vi "ICRA2024测试椭圆分裂 - 副本.vi"() -> ()   [LabVIEW 2018]
doc: "Demonstrates the use of the Network Streams functions to send LED status to the myRIO target."
uses:
  <vilib>/vision/Contour.llb/IMAQ Contour Curve Extraction.ctl
  <vilib>/ErrorRing/Error Ring.xnode
  <vilib>/vision/NI_Vision_Development_Module.lvlib
panel:
  out "len3":dbl
  out "len2":dbl
  out "len1":dbl
  out "len0":dbl
  out "Y4":sgl
  out "Y3":sgl
  out "Y2":sgl
  out "Y1":sgl
  out "Y0":sgl
  in  "Search Rect (entire image)":T1={"Left"=200, "Top"=120, "Right"=2000, "Bottom"=1920, "Rotation"=0.0} {"Rotation" format="%.2f"; "Left" scale=0.0..1024.0; "Right" scale=0.0..1024.0}
  out "长度":dbl
  out "备用的椭圆角度":sgl
  in  "打开轨迹":bool
  out "Image 9":T2(plugin-control)
  in  "Search Direction":T3(ring)
  in  "Contour Selection":T4(ring)
  in  "Number of Erosion":i32=10
  in  "椭圆磁场开关":bool=TRUE
  out "Image 7":T2(plugin-control)
  out "Ellipse":T5 {"Center"."Y" format="%.2f"; "Center"."X" format="%.2f"}
  out "Image 5":T2(plugin-control)
  in  "Contour Points Settings":T6={"Overlay?"=FALSE, "Color"=16711680, "Width"=1, "Maintain Width?"=TRUE}
  in  "Contour Equation Settings":T6={"Overlay?"=TRUE, "Color"=3381759, "Width"=1, "Maintain Width?"=TRUE}
  out "ROI Descriptor Out":T7 {"Contours"."Type" items=["No Selection", "Point", "Line", "Rectangle", "Oval", "Polygon", "Freehand Region", "Annulus", "Unused2", "Unused3", "Broken Line", "Freehand Line", "Rotated Rectangle"]}
  in  "Curve Extraction":T8={"Extraction Mode"=0, "Edge Threshold"=75, "Edge Filter Size"=1, "Min Length"=25, "Search Step Size"=15, "Max Endpoint Gap"=10, "Subpixel"=TRUE} {"Extraction Mode" items=["Normal", "Uniform Regions"]; "Edge Filter Size" items=["Fine", "Normal", "Contour Tracing"]; "Max Endpoint Gap" min=0; "Search Step Size" min=1 max=255 step=1; "Min Length" min=0; "Edge Threshold" min=1 max=350 step=1}
  out "Image 4":T2(plugin-control)
  out "Image":T2(plugin-control)
  in  "Acquisition Control::Acquisition Frame Rate":dbl=19.50304412841797 min=1.4211589097976685 max=44.94382095336914
  out "Stopped":bool
  in  "Stop (F) 2":bool caption="Stop (F)"
  out "Objects 2":T9(array[cluster]) {"Aspect Ratio" format="%.2f"; "Orientation" format="%.2f"; "Area" format="%.2f"; "Object Center"."Y" format="%.2f"; "Object Center"."X" format="%.2f"}
  in  "Settings 2":T10={"Objects"=0, "Threshold"=128, "Reject Border"=FALSE, "Fill Holes"=FALSE, "Min Object Size"=TRUE, "Min Size"=20000, "Max Object Size"=FALSE, "Max Size"=100, "Show Search Area"=FALSE, "Show Center"=TRUE, "Show Bounding Box"=TRUE} {"Objects" items=["Bright Objects", "Dark Objects"]; "Threshold" min=1 max=999999999 step=1; "Max Size" min=1 max=999999999 step=1; "Min Size" min=1 max=999999999 step=1}
  in  "Range 2":cluster{"Lower value":sgl, "Upper value":sgl}={"Lower value"=0.0, "Upper value"=230.0} {"Upper value" format="%.2f"; "Lower value" format="%.2f"}
  in  "Pause":bool
  out "Array":dbl[](array[numeric])
  in  "Parameter Settings":T11(tab)=enum."Ribbon Oscillating Field" caption="Field Types"
  in  "fg":dbl
  in  "pg":dbl
  in  "dg":dbl
  in  "Ag":dbl
  in  "AoOF":dbl
  in  "fo":sgl
  in  "do":sgl
  in  "oo":sgl
  in  "po":sgl
  in  "cc":sgl
  in  "pc":sgl
  in  "wc":sgl
  in  "dc":sgl
  in  "Ac":dbl
  in  "pr":sgl
  in  "Ar":dbl=8.0
  in  "wr":sgl=18.0
  in  "dr":sgl
  in  "Dis phase step":dbl
  in  "Dis phase frequency (Hz)":dbl
  in  "Dis tumbling frequency (Hz)":dbl
  in  "Dis strength(mT)":dbl
  in  "Swa strength (mT)":dbl
  in  "Swa frequency (Hz)":dbl
  in  "Swa pitch angle (deg)":dbl
  in  "Swa direction angle (deg)":dbl
  in  "Swa ratio":dbl=1.0
  in  "Pitch Angle (rotating around Constant, deg)":dbl
  in  "Ratio (A/C)":sgl=3.0
  in  "Direction Angle (deg)":sgl=90.0
  in  "Pitch Angle (rotating around Origin, deg)":sgl
  in  "Frequency (Hz)":sgl=6.0
  in  "Strength (mT)":dbl=3.0
  in  "Ar 2":dbl=5.0 caption="Ar"
  in  "ratio":sgl=1.0
  in  "运动方向":sgl
  in  "长轴方向":sgl
  in  "wr  2":sgl=8.0
  in  "速度大小":sgl
  out "Angle":dbl
  out "aspect ratio":dbl
  out "时间":i32
  out "Numeric 5":i32
  in  "Stop":bool
  out "error out":errorcluster
  in  "Target IP Address":string="172.22.11.2"
  # "Overview: Magnetic field calculation, and send parameters to myRIO\nInstructions:\n1. Verify the value of Target IP Address. Set Visa resource name.\n2. Ensure RT Main.vi is already running. \n3. Run this VI. Set parameters of magnetic field."
  # "Strength (mT)"
  # "Pitch Angle (deg)"
  # "Direction Angle (deg)"
  # "Frequency (Hz)"
  # "Strength (mT)"
  # "Oscilation Frequency (Hz)"
  # "Oscilation Angle (deg)"
  # "Pitch Angle (deg)"
  # "Direction Angle (deg)"
  # "Strength (mT)"
  # "Frequency (Hz)"
  # "Pitch Angle (deg)"
  # "Direction Angle (deg)"
  # "Conical Angle (deg)"
  # "Strength (mT)"
  # "Frequency (Hz)"
  # "Pitch Angle (deg)"
  # "Direction Angle (deg)"
  # "Strength (mT)"
  # "Tumbling Frequency (Hz)"
  # "Phase Frequency (Hz)"
  # "Phase Step"
  # "Strength (mT)"
  # "Frequency (Hz)"
  # "Pitch Angle (deg)"
  # "Direction Angle (deg)"
  # "Ratio"
  # "Strength (mT)"
  # "Frequency (Hz)"
  # "Ratio (A/C)"
  # "Direction Angle (deg)"
  # "Pitch Angle (rotating around Origin, deg)"
  # "Pitch Angle (rotating around Constant, deg)"
  # "Strength (mT)"
  # "Frequency (Hz)"
  # "Pitch Angle  (deg)"
  # "longaxis"
  # "Direction Angle (deg)"
  # "ratio (l/s)"
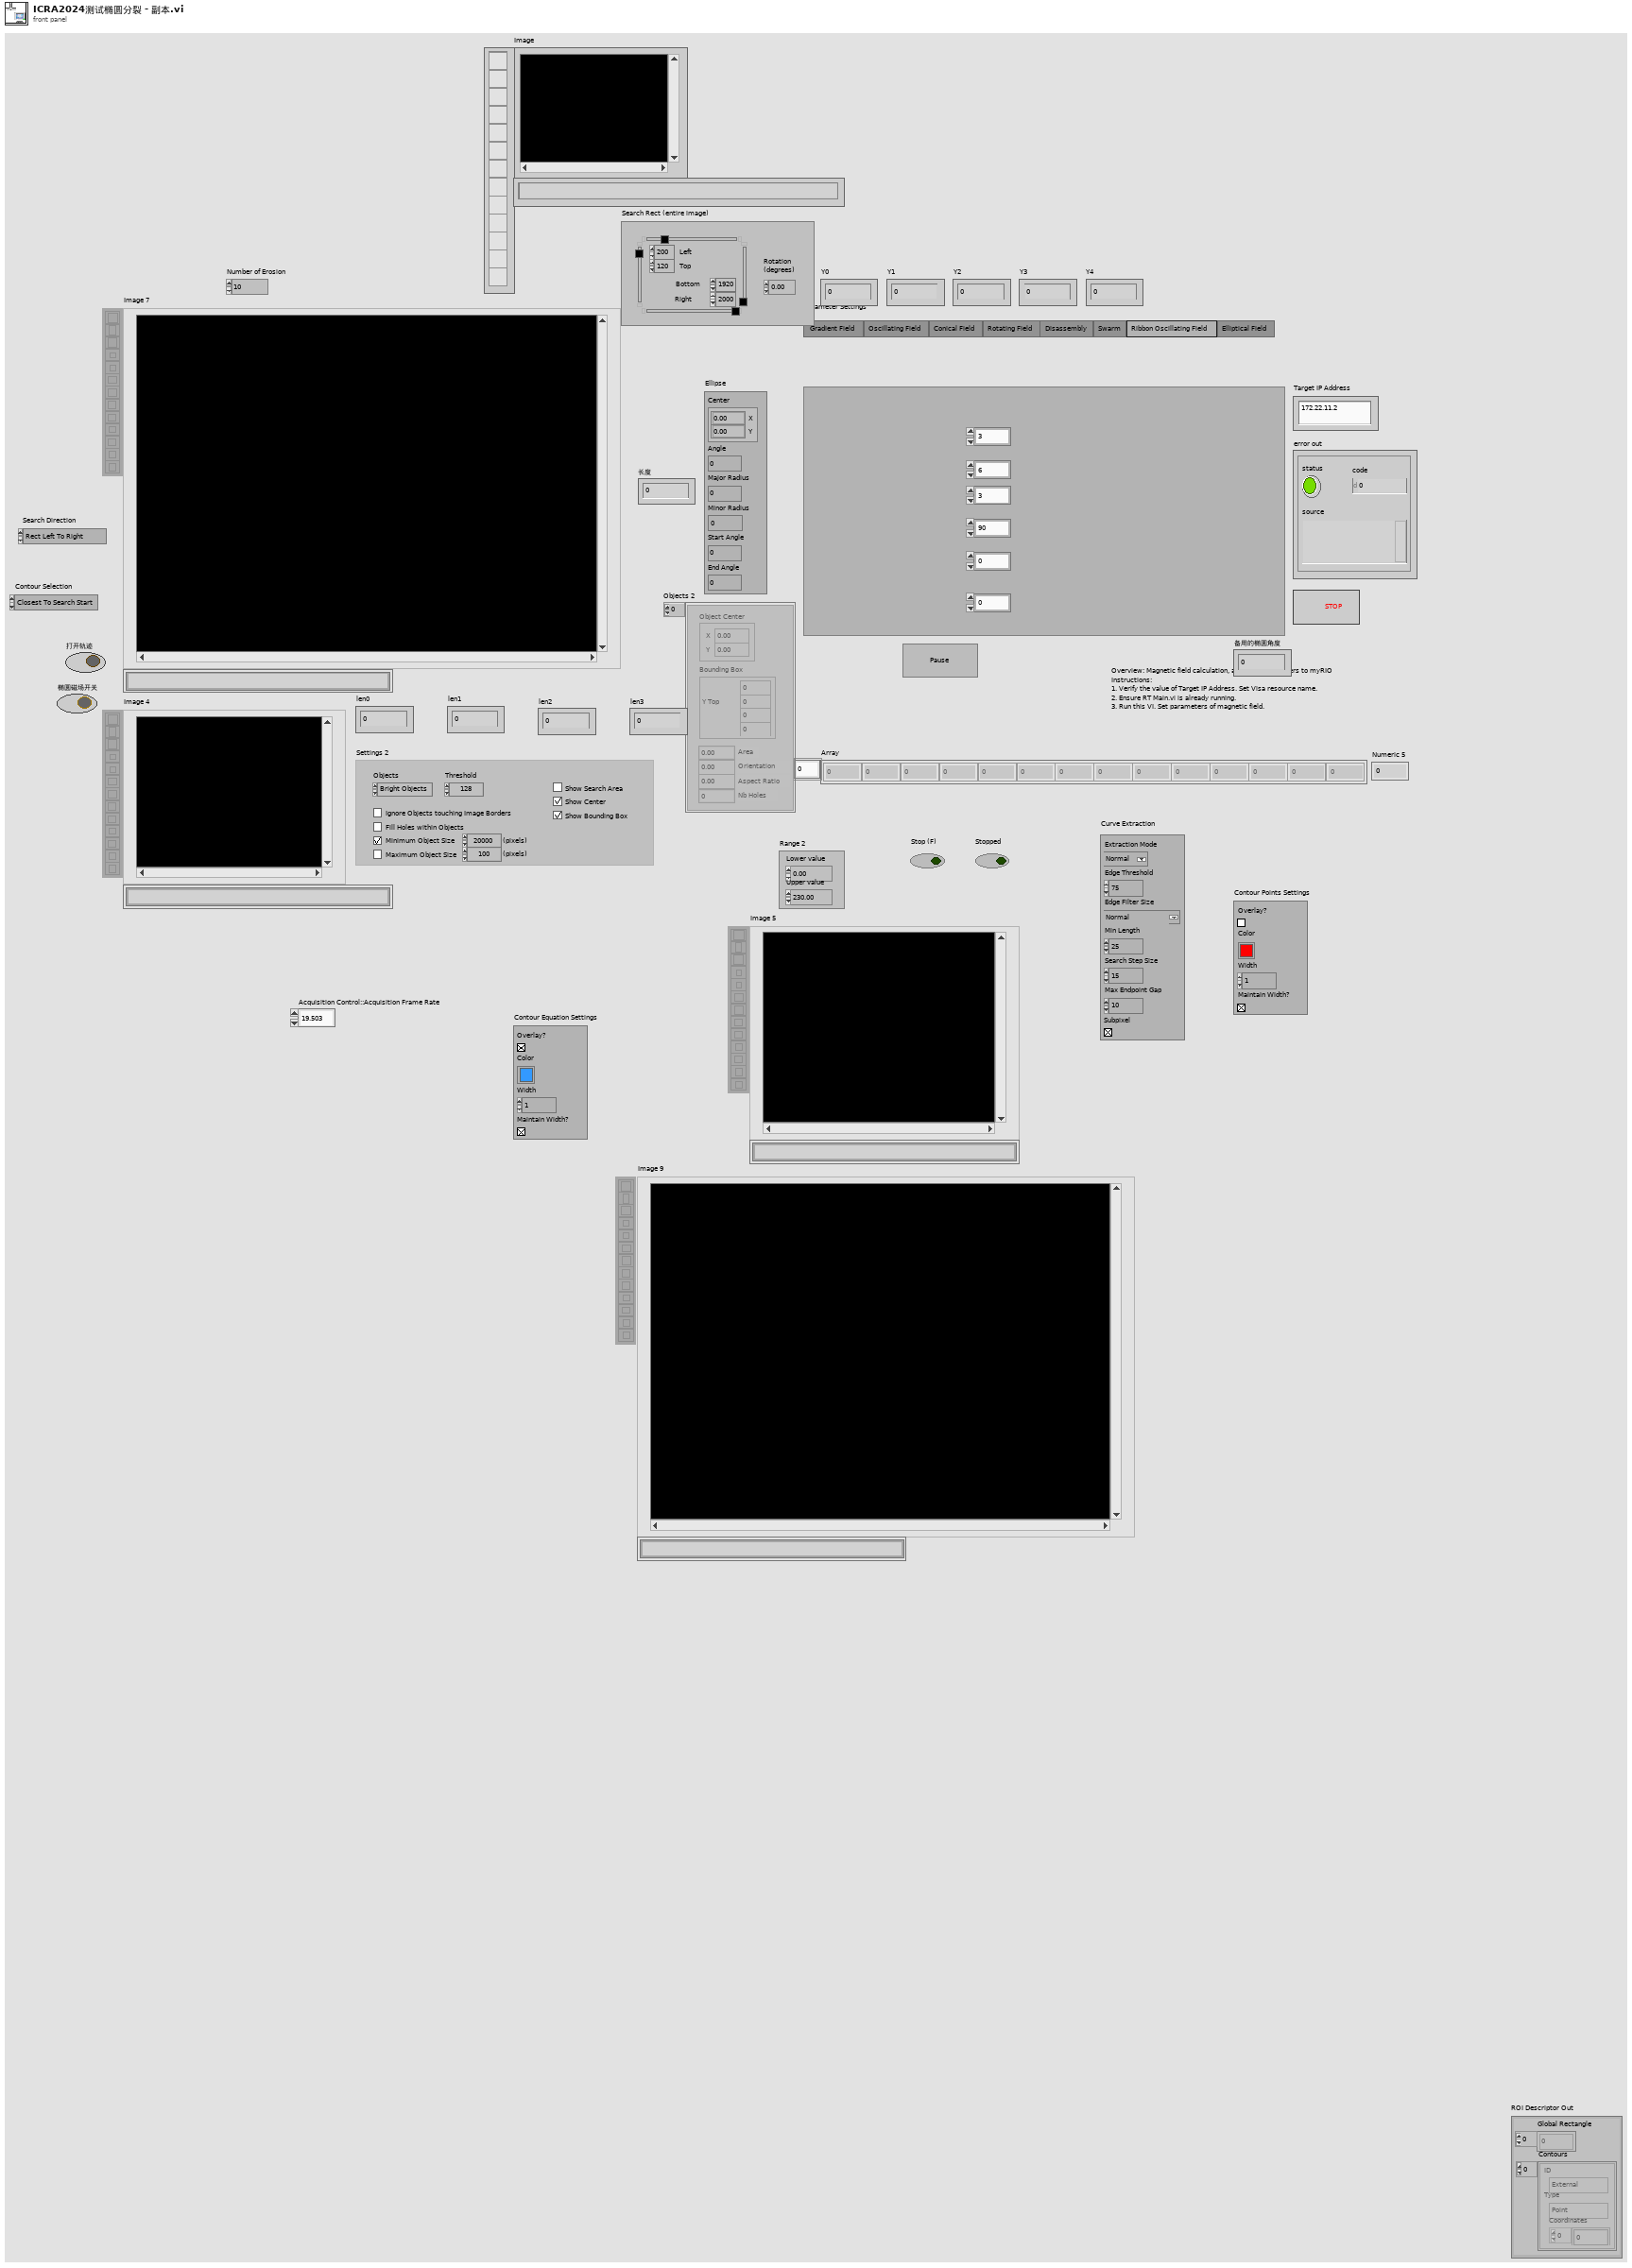
[diagram p1: front panel]
types:
  T1 = typedef "IMAQ Rectangle" = cluster{"Left":i32, "Top":i32, "Right":i32, "Bottom":i32, "Rotation":dbl}
  T2 = typedef "IMAQ Image.ctl" = refnum<image>
  T3 = enum16{"Rect Left To Right", "Rect Right To Left", "Rect Top To Bottom", "Rect Bottom To Top", "Annulus Inner To Outer", "Annulus Outer To Inner", "Annulus Start Angle To End Angle", "Annulus End Angle To Start Angle"}
  T4 = enum16{"Closest To Search Start", "Maximum Length", "Strongest Mean Gradient Change"}
  T5 = cluster{"Center":cluster{"X":sgl, "Y":sgl}, "Angle":dbl, "Major Radius":dbl, "Minor Radius":dbl, "Start Angle":dbl, "End Angle":dbl}
  T6 = cluster{"Overlay?":bool, "Color":u32, "Width":u32, "Maintain Width?":bool}
  T7 = typedef "ROI Descriptor" = cluster{"Global Rectangle":i32[], "Contours":cluster{"ID":enum32{"External", "Internal"}, "Type":u32, "Coordinates":i32[]}[]}
  T8 = typedef "IMAQ Contour Curve Extraction.ctl" = cluster{"Extraction Mode":u32, "Edge Threshold":i32, "Edge Filter Size":u32, "Min Length":i32, "Search Step Size":i32, "Max Endpoint Gap":i32, "Subpixel":bool}
  T9 = cluster{"Object Center":cluster{"X":sgl, "Y":sgl}, "Bounding Box":cluster{"X Left":i32, "Y Top":i32, "X Right":i32, "Y Bottom":i32}, "Area":sgl, "Orientation":sgl, "Aspect Ratio":sgl, "Nb Holes":i32}[]
  T10 = cluster{"Objects":u16, "Threshold":i32, "Reject Border":bool, "Fill Holes":bool, "Min Object Size":bool, "Min Size":i32, "Max Object Size":bool, "Max Size":i32, "Show Search Area":bool, "Show Center":bool, "Show Bounding Box":bool}
  T11 = enum32{"Gradient Field ", "Oscillating Field", "Conical Field", "Rotating Field", "Disassembly", "Swarm", "Ribbon Oscillating Field", "Elliptical Field"}
  T12 = enum32{"AutoM", "Close", "Dilate", "Erode", "Gradient", "Gradient in", "Gradient out", "HitMiss", "Open", "PClose", "POpen", "Thick", "Thin"}
  T13 = typedef "Image Type" = u32
  T14 = cluster{"Objects[0]":cluster{"Object Center":cluster{"X":sgl, "Y":sgl}, "Bounding Box":cluster{"X Left":i32, "Y Top":i32, "X Right":i32, "Y Bottom":i32}, "Area":sgl, "Orientation":sgl, "Aspect Ratio":sgl, "Nb Holes":i32}, "Objects[1]":cluster{"Object Center":cluster{"X":sgl, "Y":sgl}, "Bounding Box":cluster{"X Left":i32, "Y Top":i32, "X Right":i32, "Y Bottom":i32}, "Area":sgl, "Orientation":sgl, "Aspect Ratio":sgl, "Nb Holes":i32}, "Objects[2]":cluster{"Object Center":cluster{"X":sgl, "Y":sgl}, "Bounding Box":cluster{"X Left":i32, "Y Top":i32, "X Right":i32, "Y Bottom":i32}, "Area":sgl, "Orientation":sgl, "Aspect Ratio":sgl, "Nb Holes":i32}, "Objects[3]":cluster{"Object Center":cluster{"X":sgl, "Y":sgl}, "Bounding Box":cluster{"X Left":i32, "Y Top":i32, "X Right":i32, "Y Bottom":i32}, "Area":sgl, "Orientation":sgl, "Aspect Ratio":sgl, "Nb Holes":i32}, "Objects[4]":cluster{"Object Center":cluster{"X":sgl, "Y":sgl}, "Bounding Box":cluster{"X Left":i32, "Y Top":i32, "X Right":i32, "Y Bottom":i32}, "Area":sgl, "Orientation":sgl, "Aspect Ratio":sgl, "Nb Holes":i32}, "Objects[5]":cluster{"Object Center":cluster{"X":sgl, "Y":sgl}, "Bounding Box":cluster{"X Left":i32, "Y Top":i32, "X Right":i32, "Y Bottom":i32}, "Area":sgl, "Orientation":sgl, "Aspect Ratio":sgl, "Nb Holes":i32}, "Objects[6]":cluster{"Object Center":cluster{"X":sgl, "Y":sgl}, "Bounding Box":cluster{"X Left":i32, "Y Top":i32, "X Right":i32, "Y Bottom":i32}, "Area":sgl, "Orientation":sgl, "Aspect Ratio":sgl, "Nb Holes":i32}, "Objects[7]":cluster{"Object Center":cluster{"X":sgl, "Y":sgl}, "Bounding Box":cluster{"X Left":i32, "Y Top":i32, "X Right":i32, "Y Bottom":i32}, "Area":sgl, "Orientation":sgl, "Aspect Ratio":sgl, "Nb Holes":i32}, "Objects[8]":cluster{"Object Center":cluster{"X":sgl, "Y":sgl}, "Bounding Box":cluster{"X Left":i32, "Y Top":i32, "X Right":i32, "Y Bottom":i32}, "Area":sgl, "Orientation":sgl, "Aspect Ratio":sgl, "Nb Holes":i32}}
  T15 = cluster{"Object Center":cluster{"X":sgl, "Y":sgl}, "Bounding Box":cluster{"X Left":i32, "Y Top":i32, "X Right":i32, "Y Bottom":i32}, "Area":sgl, "Orientation":sgl, "Aspect Ratio":sgl, "Nb Holes":i32}
  T16 = cluster{"X Left":i32, "Y Top":i32, "X Right":i32, "Y Bottom":i32}
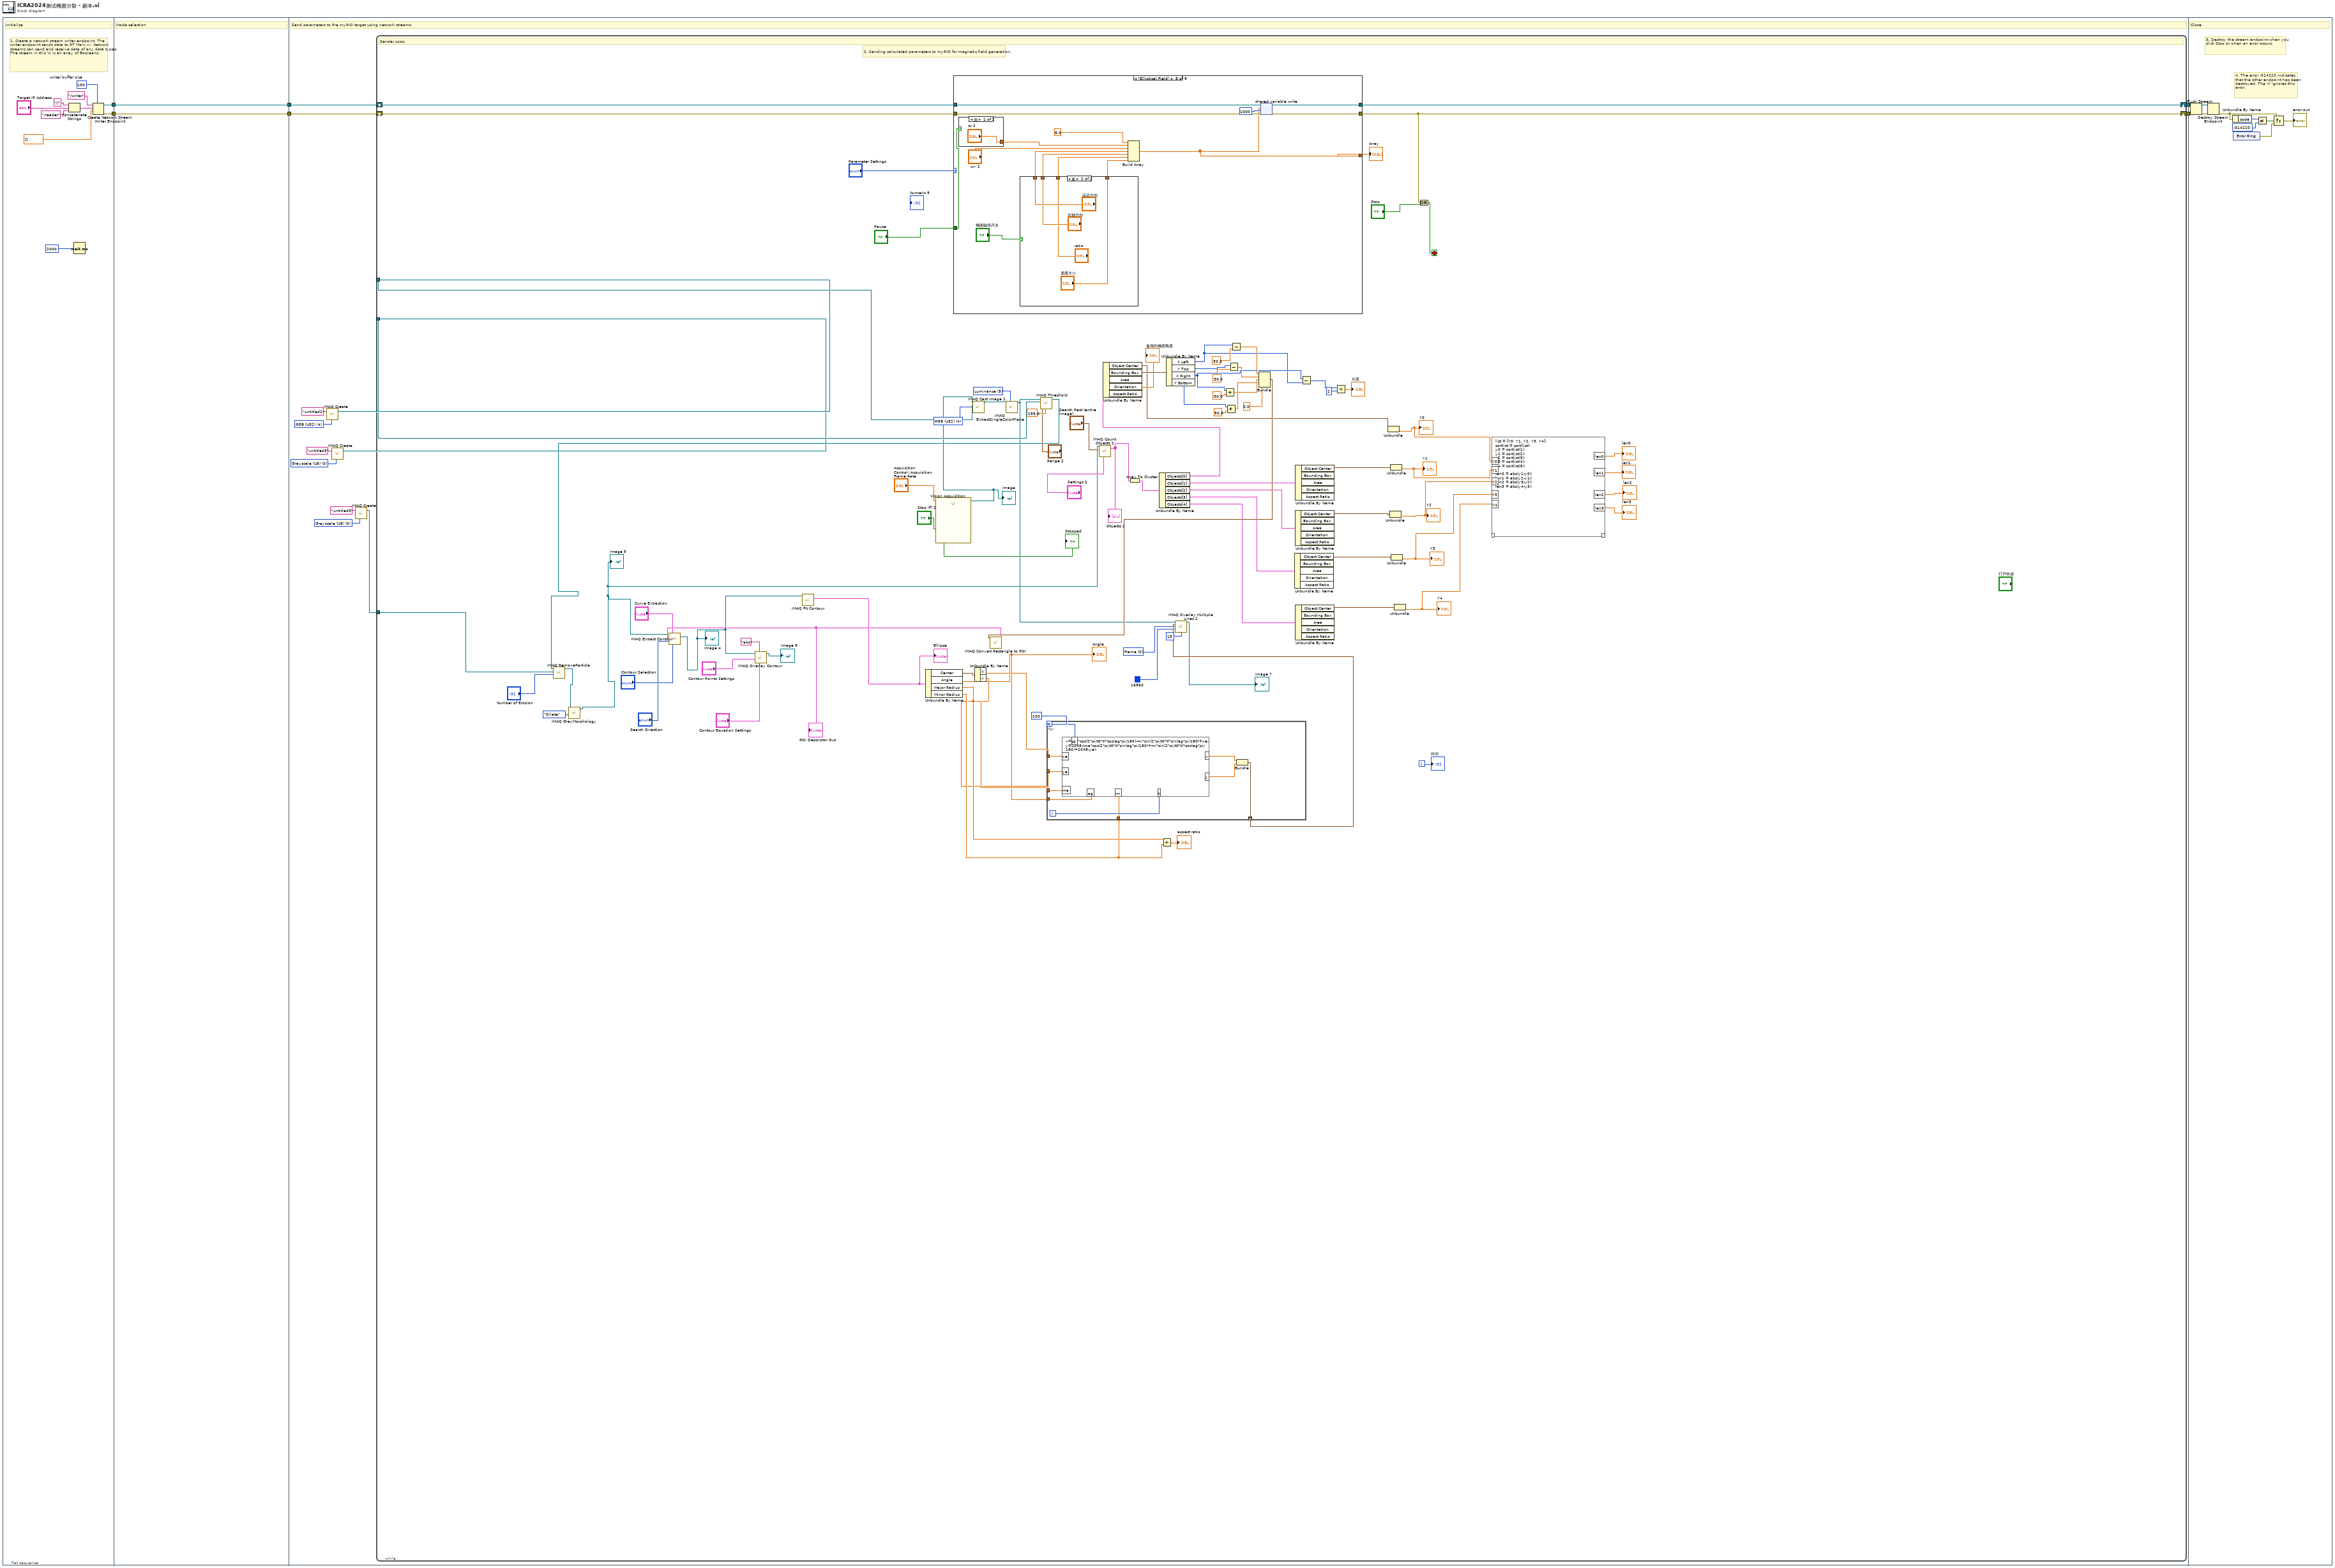
[diagram p0: block diagram]
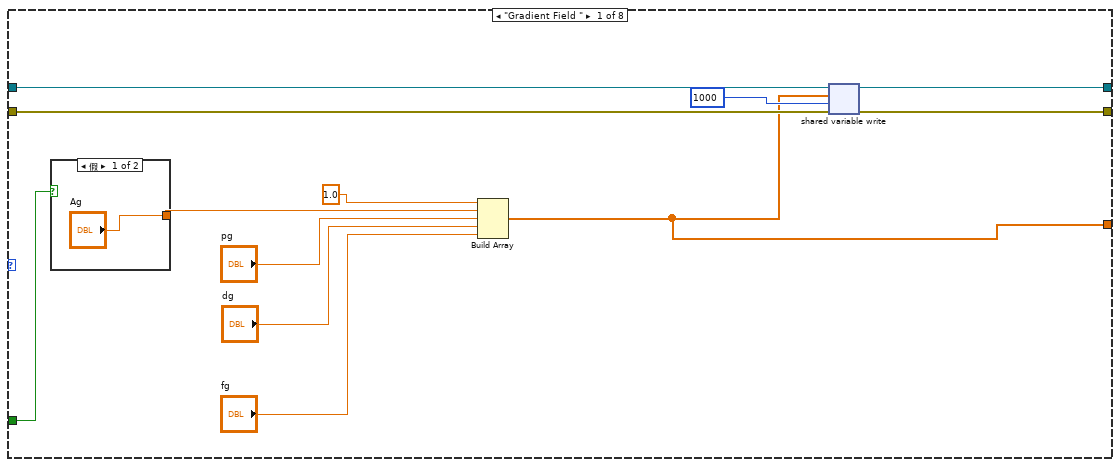
[diagram p2: hidden frame]
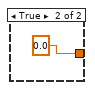
[diagram p3: hidden frame]
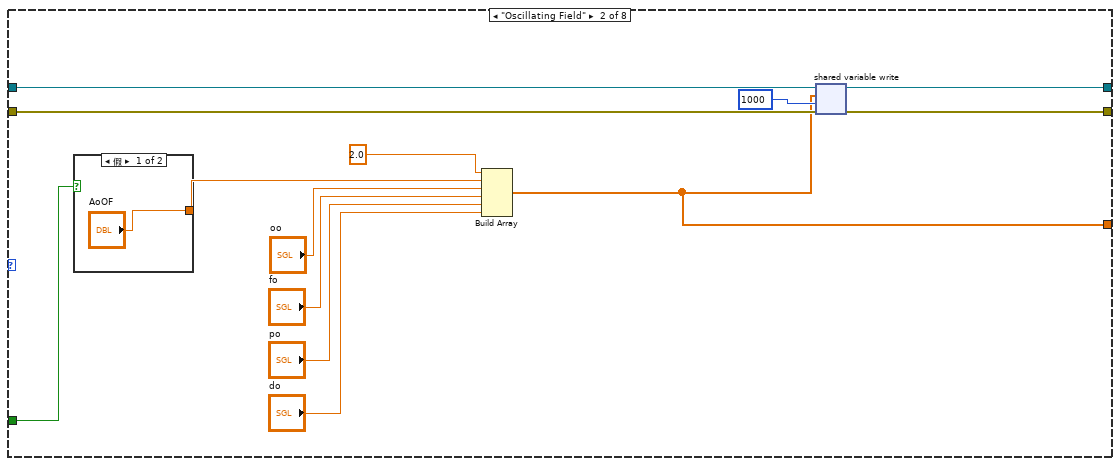
[diagram p4: hidden frame]
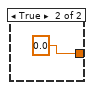
[diagram p5: hidden frame]
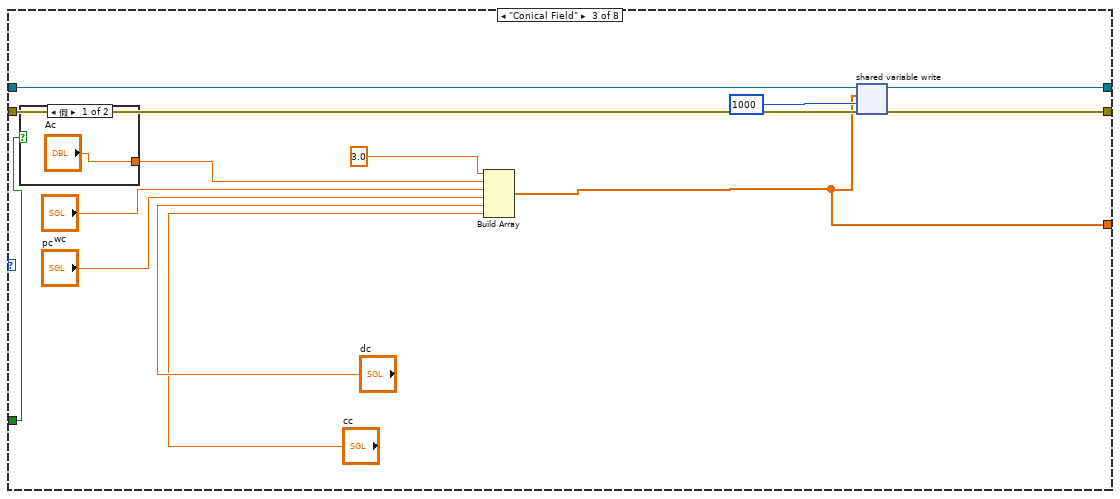
[diagram p6: hidden frame]
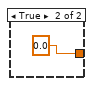
[diagram p7: hidden frame]
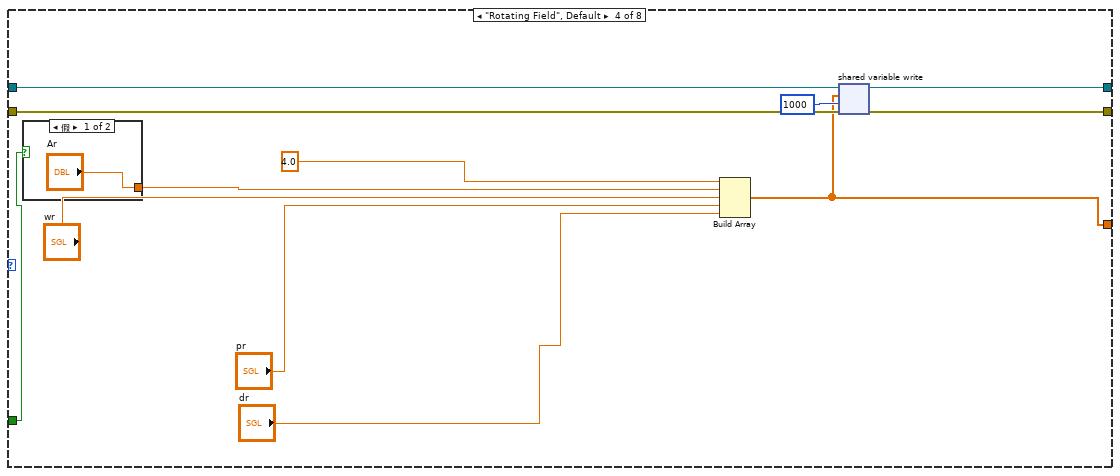
[diagram p8: hidden frame]
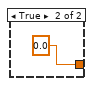
[diagram p9: hidden frame]
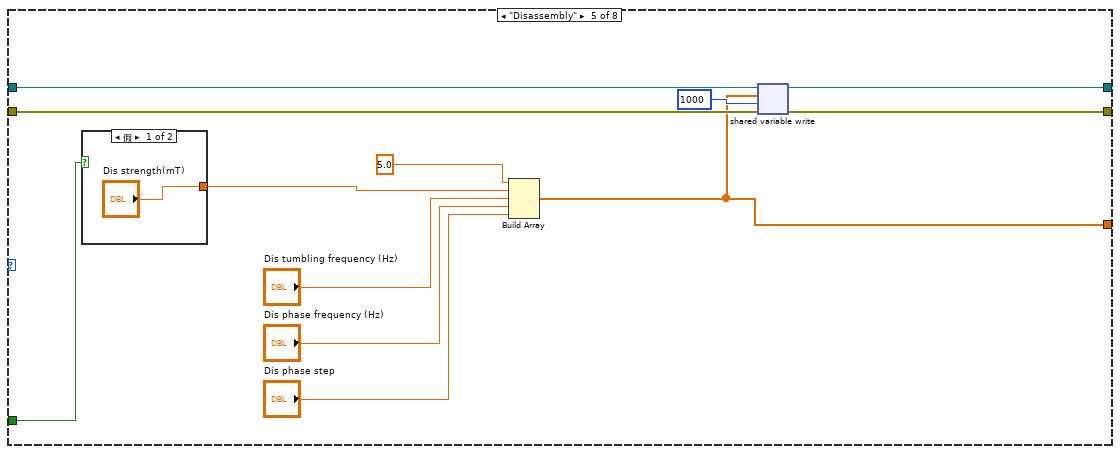
[diagram p10: hidden frame]
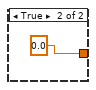
[diagram p11: hidden frame]
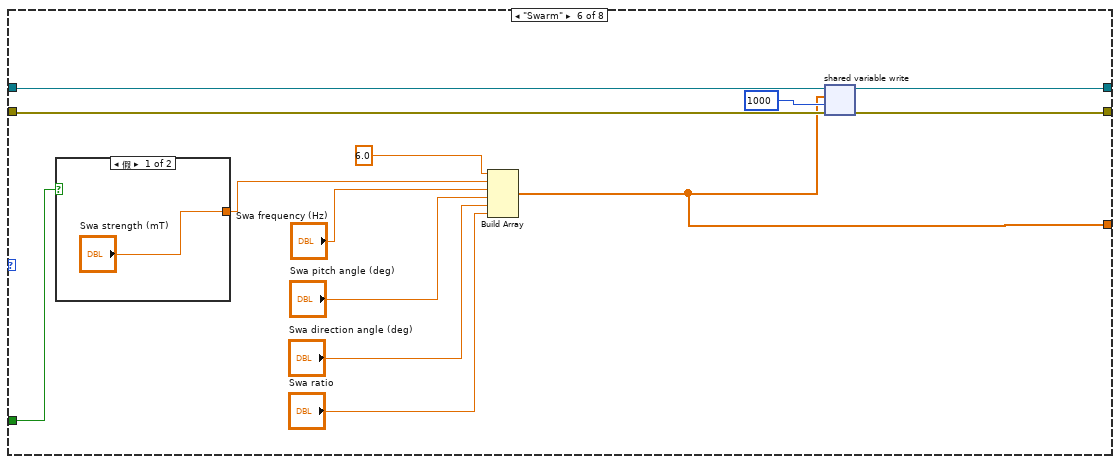
[diagram p12: hidden frame]
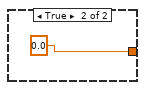
[diagram p13: hidden frame]
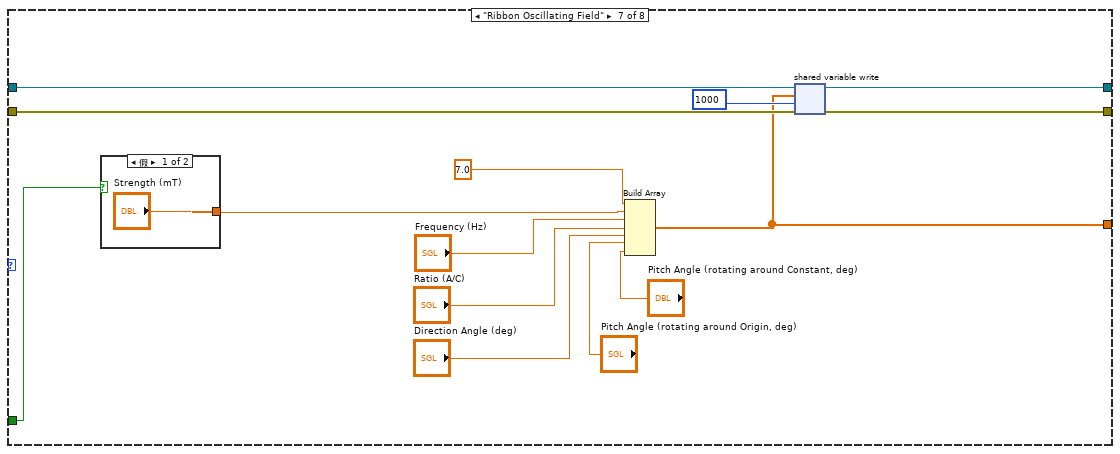
[diagram p14: hidden frame]
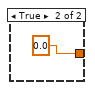
[diagram p15: hidden frame]
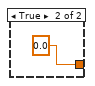
[diagram p17: hidden frame]
diagram:
  n1 = flat-sequence {
    tunnel: [w11] -> w2
    tunnel: [w10] -> w1
    tunnel: [w18] -> w4
    tunnel: [w17] -> w3
    tunnel: w1 -> [w17]
    tunnel: w2 -> [w18]
    tunnel: [w29] -> w6
    tunnel: w4 -> [w31]
    tunnel: [w28] -> w5
    tunnel: w3 -> [w30]
    tunnel: w6 -> [w268]
    tunnel: w5 -> [w265]
    frame #0 {
      w9 = 100  # writer buffer size
      # "1. Create a network stream writer endpoint. The writer endpoint sends data to RT Main.vi. Network streams can send and receive data of any data types. The stream in this VI is an array of Booleans."
      # "Initialize"
      n2 = Concatenate Strings("//", "Target IP Address", "/reader") -> (w16:string)
      n3 = Wait (ms)(milliseconds to wait=2000) -> ()  [unwired: 1 out]
      n4 = Create Network Stream Writer Endpoint(7:w9, 9:dbl[] [], 10:w16, 11:"/writer" ("reader name")) -> (0:w10:errorcluster, 3:w11:refnum<k21>)  [unwired: 3 in]
    }
    frame #1 {
      # "Mode selection"
    }
    frame #2 {
      w20 = T13 0 items=["Grayscale (U8)", "Grayscale (I16)", "Grayscale (SGL)", "Complex (CSG)", "RGB (U32)", "HSL (U32)", "RGB (U64)", "Grayscale (U16)"] ("Image Type")
      w24 = T13 0 items=["Grayscale (U8)", "Grayscale (I16)", "Grayscale (SGL)", "Complex (CSG)", "RGB (U32)", "HSL (U32)", "RGB (U64)", "Grayscale (U16)"] ("Image Type")
      w26 = T13 4 items=["Grayscale (U8)", "Grayscale (I16)", "Grayscale (SGL)", "Complex (CSG)", "RGB (U32)", "HSL (U32)", "RGB (U64)", "Grayscale (U16)"] ("Image Type")
      # "Send parameters to the myRIO target using network streams"
      n5 = call "IMAQ Create"("Image Name"="untitled2", "Image Type"=w26) -> ("New Image"=w23:T2)  [unwired: 3 in, 1 out]
      n6 = call "IMAQ Create"("Image Name"="untitled3", "Image Type"=w24) -> ("New Image"=w22:T2)  [unwired: 3 in, 1 out]
      n7 = call "IMAQ Create"("Image Name"="untitled3", "Image Type"=w20) -> ("New Image"=w19:T2)  [unwired: 3 in, 1 out]
      n8 = while {
        shift-right: [w120] -> w28
        shift-left: w30 -> [w122]
        shift-right: [w121] -> w29
        shift-left: w31 -> [w123]
        tunnel: w22 -> [w111]
        tunnel: w23 -> [w106]
        tunnel: w19 -> [w74]
        i -> [w57]
        stop <- w110 stop-if-true
        w93 = u32 0 items=["Frame", "Fill"] ("Drawing Mode (Frame)")
        w105 = T13 4 items=["Grayscale (U8)", "Grayscale (I16)", "Grayscale (SGL)", "Complex (CSG)", "RGB (U32)", "HSL (U32)", "RGB (U64)", "Grayscale (U16)"] ("Image Type")
        w116 = 5 items=["Red", "Green", "Blue", "Hue", "Saturation", "Luminance", "Value", "Intensity"] ("Color Plane")
        # "2. Sending calculated parameters to myRIO for magnetic field generation."
        # "Sender Loop"
        n9 = call "Vision Acquisition"("Acquisition Control::Acquisition Frame Rate"="Acquisition Control::Acquisition Frame Rate", "Stop (F)"="Stop (F) 2") -> ("Image Out"=w104:T2, "Stopped"=→"Stopped":bool)  [unwired: 23 in, 1 out]
        "Image" <- w104
        n10 = case shown="\"Elliptical Field\"" "Parameter Settings" {
          tunnel: w123 -> [w145 w160 w175 w189 w203 w217 w235 w251]
          tunnel: w122 -> [w142 w159 w174 w188 w201 w216 w233 w250]
          tunnel: [w144 w158 w172 w187 w202 w215 w234 w249] -> w121
          tunnel: [w143 w157 w173 w186 w200 w214 w232 w248] -> w120
          tunnel: [w138 w151 w166 w181 w194 w209 w230 w243] -> w119
          tunnel: "Pause" -> [w136 w149 w164 w179 w193 w208 w225 w241]
          frame "Gradient Field " {
            n11 = case shown="假" w136 {
              tunnel: ["Ag" 0.0] -> w137
              frame False {
              }
              frame True {
              }
            }
            n12 = Build Array(1.0, w137, "pg", "dg", "fg") -> (w138:dbl[])
            n13 = shared-variable-write(w145, w142, w138, 1000 ("timeout ms (-1)")) -> (w144:refnum<k21>, w143:errorcluster)  [unwired: 1 out]
          }
          frame "Oscillating Field" {
            n14 = case shown="假" w149 {
              tunnel: ["AoOF" 0.0] -> w150
              frame False {
              }
              frame True {
              }
            }
            n15 = Build Array(2.0, w150, "oo", "fo", "po", "do") -> (w151:dbl[])
            n16 = shared-variable-write(w160, w159, w151, 1000 ("timeout ms (-1)")) -> (w158:refnum<k21>, w157:errorcluster)  [unwired: 1 out]
          }
          frame "Conical Field" {
            # "FG"
            n17 = case shown="假" w164 {
              tunnel: ["Ac" 0.0] -> w165
              frame False {
              }
              frame True {
              }
            }
            n18 = Build Array(3.0, w165, "wc", "pc", "dc", "cc") -> (w166:dbl[])
            n19 = shared-variable-write(w175, w174, w166, 1000 ("timeout ms (-1)")) -> (w172:refnum<k21>, w173:errorcluster)  [unwired: 1 out]
          }
          frame "Rotating Field", Default {
            n20 = case shown="假" w179 {
              tunnel: ["Ar" 0.0] -> w180
              frame False {
              }
              frame True {
              }
            }
            n21 = Build Array(4.0, w180, "wr", "pr", "dr") -> (w181:dbl[])
            n22 = shared-variable-write(w189, w188, w181, 1000 ("timeout ms (-1)")) -> (w187:refnum<k21>, w186:errorcluster)  [unwired: 1 out]
          }
          frame "Disassembly" {
            n23 = case shown="假" w193 {
              tunnel: ["Dis strength(mT)" 0.0] -> w198
              frame False {
              }
              frame True {
              }
            }
            n24 = Build Array(5.0, w198, "Dis tumbling frequency (Hz)", "Dis phase frequency (Hz)", "Dis phase step") -> (w194:dbl[])
            n25 = shared-variable-write(w203, w201, w194, 1000 ("timeout ms (-1)")) -> (w202:refnum<k21>, w200:errorcluster)  [unwired: 1 out]
          }
          frame "Swarm" {
            n26 = case shown="假" w208 {
              tunnel: ["Swa strength (mT)" 0.0] -> w207
              frame False {
              }
              frame True {
              }
            }
            n27 = Build Array(6.0, w207, "Swa frequency (Hz)", "Swa pitch angle (deg)", "Swa direction angle (deg)", "Swa ratio") -> (w209:dbl[])
            n28 = shared-variable-write(w217, w216, w209, 1000 ("timeout ms (-1)")) -> (w215:refnum<k21>, w214:errorcluster)  [unwired: 1 out]
          }
          frame "Ribbon Oscillating Field" {
            n29 = case shown="假" w225 {
              tunnel: ["Strength (mT)" 0.0] -> w224
              frame False {
              }
              frame True {
              }
            }
            n30 = Build Array(7.0, w224, "Frequency (Hz)", "Ratio (A/C)", "Direction Angle (deg)", "Pitch Angle (rotating around Origin, deg)", "Pitch Angle (rotating around Constant, deg)") -> (w230:dbl[])
            n31 = shared-variable-write(w235, w233, w230, 1000 ("timeout ms (-1)")) -> (w234:refnum<k21>, w232:errorcluster)  [unwired: 1 out]
          }
          frame "Elliptical Field" {
            n32 = case shown="假" w241 {
              tunnel: ["Ar 2" 0.0] -> w242
              frame False {
              }
              frame True {
              }
            }
            n33 = case shown="真" "椭圆磁场开关" {
              tunnel: [_ "运动方向"] -> w246
              tunnel: [_ "长轴方向"] -> w245
              tunnel: [_ "ratio"] -> w240
              tunnel: [_ "速度大小"] -> w239
              frame False {
              }
              frame True {
              }
            }
            n34 = Build Array(8.0, w242, "wr  2", w246, w245, w240, w239) -> (w243:dbl[])
            n35 = shared-variable-write(w251, w250, w243, 1000 ("timeout ms (-1)")) -> (w249:refnum<k21>, w248:errorcluster)  [unwired: 1 out]
          }
        }
        "Array" <- w119
        n36 = call "IMAQ Cast Image 2"("Image Src"=w104, "Image Dst"=w106, "Image Type"=w105) -> ("Image Dst Out"=w107:T2)  [unwired: 11 in, 1 out]
        n37 = call "IMAQ ExtractSingleColorPlane"("Color Plane"=w116, "Image Src"=w107) -> ("Image Dst Out"=w66:T2)  [unwired: 8 in, 1 out]
        n38 = call "IMAQ Threshold"("Replace Value"=sgl 255.0, "Range"="Range 2", "Image Dst"=w111, "Image Src"=w66) -> ("Image Dst Out"=w75:T2)  [unwired: 6 in, 1 out]
        n39 = call "IMAQ RemoveParticle"("Number of Erosion"="Number of Erosion", "Image Dst"=w74, "Image Src"=w75) -> ("Image Dst Out"=w70:T2)  [unwired: 7 in, 1 out]
        n40 = call "IMAQ GrayMorphology"("Operation"=T12."Dilate", "Image Src"=w70) -> ("Image Dst Out"=w67:T2)  [unwired: 8 in, 1 out]
        "Image 5" <- w67
        n41 = call "IMAQ Count Objects 2"("Settings"="Settings 2", "Search Rect (entire image)"="Search Rect (entire image)", "Image"=w67) -> ("Objects"=w112:T9)  [unwired: 4 in, 4 out]
        "Objects 2" <- w112
        n42 = Array To Cluster(array=w112) -> (cluster=w77:T14)
        n43 = Unbundle By Name(w77) -> ("Objects[0]"=w76:T15, "Objects[1]"=w49:T15, "Objects[2]"=w48:T15, "Objects[3]"=w47:T15, "Objects[4]"=w42:T15)
        n44 = Unbundle By Name(w76) -> ("Object Center"=w45:cluster{"X":sgl, "Y":sgl}, "Bounding Box"=w92:T16, "Orientation"=→"备用的椭圆角度":sgl)  [unwired: 2 out]
        n45 = Unbundle By Name(w92) -> ("X Left"=w54:i32, "Y Top"=w87:i32, "X Right"=w55:i32, "Y Bottom"=w86:i32)
        n46 = Add(x=w55, y=50.0) -> (x+y=w83:dbl)
        n47 = Add(x=w86, y=50.0) -> (x+y=w82:dbl)
        n48 = Subtract(x=w87, y=50.0) -> (x-y=w84:dbl)
        n49 = Subtract(x=w54, y=50.0) -> (x-y=w85:dbl)
        n50 = Bundle(w85, w84, w83, w82, 0.0) -> (w80:cluster{dbl, dbl, dbl, dbl, dbl})  [unwired: 1 in]
        n51 = call "IMAQ Convert Rectangle to ROI"("Rectangle"=w80) -> ("ROI Descriptor"=w79:T7)  [unwired: 8 in, 1 out]
        "ROI Descriptor Out" <- w79
        n52 = call "IMAQ Extract Contour"("Source Image"=w67, "Curve Extraction"="Curve Extraction", "ROI Descriptor"=w79, "Search Direction"="Search Direction", "Contour Selection"="Contour Selection") -> ("Contour Image Out"=w99:T2)  [unwired: 6 in, 4 out]
        "Image 4" <- w99
        n53 = call "IMAQ Overlay Contour"("Contour Equation Settings"="Contour Equation Settings", "Group"="abc", "Contour Points Settings"="Contour Points Settings", "Image"=w99) -> ("Image Out"=→"Image 9":T2)  [unwired: 6 in, 1 out]
        n54 = call-poly "IMAQ Fit Contour"("Contour Image"=w99) -> ("Ellipse"=w97:T5)  [unwired: 8 in, 2 out]
        "Ellipse" <- w97
        n55 = Unbundle By Name(w97) -> ("Center"=w98:cluster{"X":sgl, "Y":sgl}, "Angle"=w61:dbl, "Major Radius"=w64:dbl, "Minor Radius"=w65:dbl)
        "Angle" <- w61
        n56 = Unbundle By Name(w98) -> ("X"=w63:sgl, "Y"=w62:sgl)
        n57 = for {
          N: 200 -> [w130]
          tunnel: [w131] -> w78 mode=indexing
          tunnel: w63 -> [w129]
          tunnel: w62 -> [w128]
          tunnel: w64 -> [w127]
          tunnel: w61 -> [w126]
          tunnel: w65 -> [w125]
          i -> [w132]
          n58 = formula code="x=ma*cos(2*pi/t0*t)*cos(ag*pi/180)-mi*sin(2*pi/t0*t)*sin(ag*pi/180)+xe;\ny=2048-(ma*cos(2*pi/t0*t)*sin(ag*pi/180)+mi*sin(2*pi/t0*t)*cos(ag*pi/180)+2048-ye);"("xe"=w129, "ye"=w128, "ma"=w127, "ag"=w126, "mi"=w125, "t"=w132, "t0"=w130) -> ("x"=w134:dbl, "y"=w133:dbl)
          n59 = Bundle("x"=w134, "y"=w133) -> (w131:cluster{"x":dbl, "y":dbl})  [unwired: 1 in]
        }
        n60 = Divide(x=w64, y=w65) -> (x/y=→"aspect ratio":dbl)
        n61 = call "IMAQ Overlay Multiple Lines 2"("Image"=w66, "Line End Points"=w78, "Drawing Mode (Frame)"=w93, "Color"=u32 16860, "Width"=u32 15) -> ("Image Out"=→"Image 7":T2)  [unwired: 9 in, 1 out]
        n62 = Unbundle By Name(w47) -> ("Object Center"=w43:cluster{"X":sgl, "Y":sgl})  [unwired: 4 out]
        n63 = Unbundle By Name(w48) -> ("Object Center"=w44:cluster{"X":sgl, "Y":sgl})  [unwired: 4 out]
        n64 = Unbundle By Name(w49) -> ("Object Center"=w46:cluster{"X":sgl, "Y":sgl})  [unwired: 4 out]
        n65 = Unbundle By Name(w42) -> ("Object Center"=w41:cluster{"X":sgl, "Y":sgl})  [unwired: 4 out]
        n66 = Subtract(x=w55, y=w54) -> (x-y=w53:i32)
        n67 = Divide(x=w53, y=2) -> (x/y=→"长度":dbl)
        n68 = Unbundle(w45) -> ("Y"=w40:sgl)  [unwired: 1 out]
        "Y0" <- w40
        n69 = Unbundle(w44) -> ("Y"=w38:sgl)  [unwired: 1 out]
        "Y2" <- w38
        n70 = Unbundle(w46) -> ("Y"=w39:sgl)  [unwired: 1 out]
        "Y1" <- w39
        n71 = Unbundle(w43) -> ("Y"=w37:sgl)  [unwired: 1 out]
        "Y3" <- w37
        n72 = Unbundle(w41) -> ("Y"=w36:sgl)  [unwired: 1 out]
        "Y4" <- w36
        n73 = Or(x=w120, y="Stop") -> (x .or. y?=w110:bool)
        n74 = script code="list = [Y0, Y1, Y2, Y3, Y4];\nsortlist = sort(list);\ny0 = sortlist(1);\ny1 = sortlist(2);\ny2 = sortlist(3);\ny3 = sortlist(4);\ny4 = sortlist(5);\n\nlen0 = abs(y1-y0);\nlen1 = abs(y2-y1);\nlen2 = abs(y3-y2);\nlen3 = abs(y4-y3);"("Y0"=w40, "Y1"=w39, "Y2"=w38, "Y3"=w37, "Y4"=w36) -> ("len0"=→"len0":dbl, "len1"=→"len1":dbl, "len2"=→"len2":dbl, "len3"=→"len3":dbl)  [unwired: 1 in, 1 out]
        "时间" <- w57
      }
    }
    frame #3 {
      # "4. The error -314220 indicates that the other endpoint has been destroyed. The VI ignores this error."
      # "3. Destroy the stream endpoint when you click Stop or when an error occurs."
      # "Close"
      n75 = Flush Stream(8:w265, 11:w268) -> (0:w266:errorcluster, 3:w267:refnum<k21>)  [unwired: 2 in, 1 out]
      n76 = Destroy Stream Endpoint(8:w266, 11:w267) -> (0:w260:errorcluster)
      n77 = Unbundle By Name(w260) -> ("code"=w264:i32)
      n78 = xnode "Error Ring"() -> ("错误输出"=w261:errorcluster)
      n79 = Not Equal?(x=w264, y=-314220) -> (x != y?=w262:bool)
      n80 = Select(t=w260, s=w262, f=w261) -> (s? t:f=→"error out":errorcluster)
    }
  }
